vi "Normalise_Signal.vi"(4 "x":dbl[](array[numeric])) -> (1 "(x-X)/sigma":dbl[](array[numeric]))   [LabVIEW 2022 SP3]
uses:
  <vilib>/Analysis/NI_AALBase.lvlib
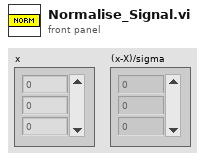
[diagram p1: front panel]
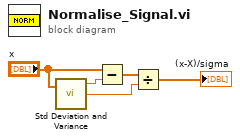
[diagram p0: block diagram]
diagram:
  n1 = call <vilib>:"Std Deviation and Variance.vi"("X"="x") -> ("mean"=w4:dbl, "standard deviation"=w2:dbl)  [unwired: 1 in, 1 out]
  n2 = Subtract(x="x", y=w4) -> (x-y=w3:dbl[])
  n3 = Divide(x=w3, y=w2) -> (x/y=→"(x-X)/sigma":dbl[])
